vi "Resize ANN configuration.vi"(1 "Configuration\nof layers":i32[](array[numeric])) -> (0 "Resized configuration\n(if necessary)":i32[](array[numeric]))   [LabVIEW 2010]
doc: "The input is an array (table) of infomation about the number of nodes in each layer. If there is an empty layer, for example: 5 4 3 0 1, this will be converted to 5 4 3."
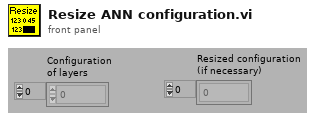
[diagram p1: front panel]
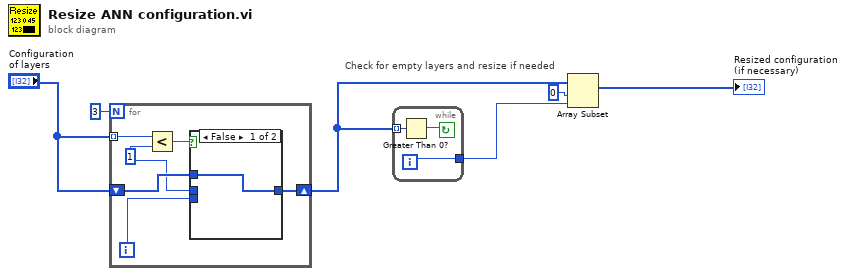
[diagram p0: block diagram]
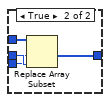
[diagram p2: hidden frame]
diagram:
  n1 = for {
    N: 3 -> [_]
    tunnel: "Configuration\nof layers" -> [w12] mode=indexing
    shift-right: [w8] -> w1
    shift-left: "Configuration\nof layers" -> [w11]
    i -> [w9]
    w10 = 1
    n2 = Less?(x=w12, y=w10) -> (x < y?=w7:bool)
    n3 = case shown="False" w7 {
      tunnel: w11 -> [w13 w17]
      tunnel: w10 -> [_ w16]
      tunnel: w9 -> [_ w15]
      tunnel: [w13 w14] -> w8
      frame False {
      }
      frame True {
        n4 = Replace Array Subset(array=w17, new element=w16, index=w15) -> (w14:i32[])
      }
    }
  }
  n5 = while "Check for empty layers and resize if needed" {
    tunnel: [w18] -> w6
    tunnel: w1 -> [w20] mode=indexing
    i -> [w18]
    stop <- w19 continue-if-true
    n6 = Greater Than 0?(x=w20) -> (x > 0?=w19:bool)
  }
  n7 = Array Subset(array=w1, index=0 ("Array Index"), length=w6) -> (→"Resized configuration\n(if necessary)":i32[])
